vi "loadImageAndConvert.vi"(8 "error in (no error)":errorcluster, 10 "name or relative path":string) -> (0 "error out":errorcluster, 2 ".NET object":refnum<k24>)   [LabVIEW 2014, in "DataGrid.lvlib" / "DataTable.lvclass"]
uses:
  DataTable.lvclass
  System.Drawing
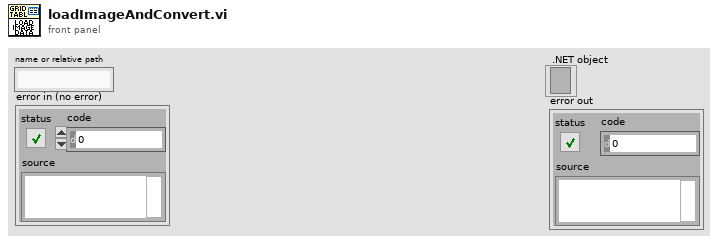
[diagram p1: front panel]
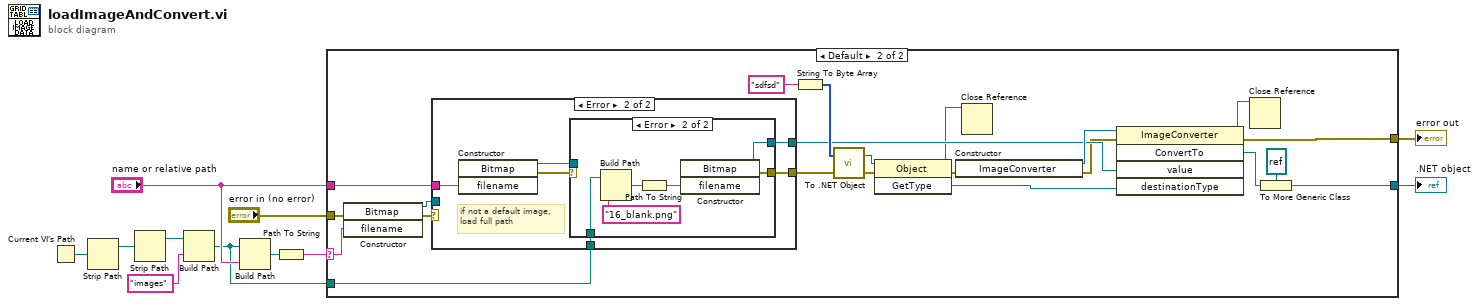
[diagram p0: block diagram]
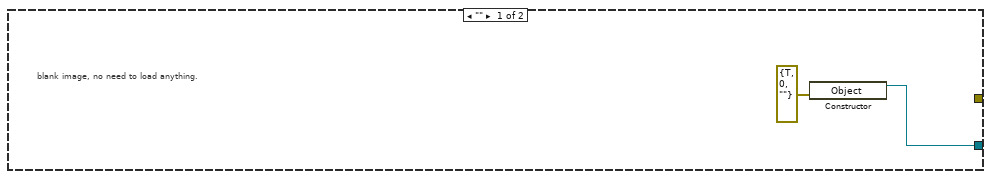
[diagram p2: hidden frame]
diagram:
  n1 = Current VI's Path() -> (path=w10:path)
  n2 = Strip Path(path=w10) -> (stripped path=w9:path)  [unwired: 1 out]
  n3 = Strip Path(path=w9) -> (stripped path=w7:path)  [unwired: 1 out]
  n4 = Build Path(base path=w7, name or relative path="images") -> (appended path=w1:path)
  n5 = Build Path(base path=w1, name or relative path="name or relative path") -> (appended path=w2:path)
  n6 = Path To String(path=w2) -> (string=w11:string)
  n7 = case shown="Default" w11 {
    selector: w11 -> [_ w35]
    tunnel: "name or relative path" -> [_ w33]
    tunnel: [w12 w16] -> w5
    tunnel: "error in (no error)" -> [_ w19]
    tunnel: [_ w15] -> w3
    tunnel: w1 -> [_ w14]
    frame "" {
      # "blank image, no need to load anything."
      n8 = constructor class="Object"(error in=errorcluster {"status"=TRUE, "code"=0, "source"=""} ("error in (no error)")) -> (reference out=w12:refnum<k24>)  [unwired: 2 in, 2 out]
    }
    frame Default {
      n9 = constructor class="Bitmap"(error in=w19, "filename"=w35) -> (reference out=w32:refnum<k24>, error out=w34:errorcluster)  [unwired: 2 in, 2 out]
      n10 = case shown="Error" w34 {
        tunnel: w33 -> [_ w42]
        tunnel: [w36 w40] -> w26
        tunnel: w32 -> [w36 _]
        tunnel: [_ w39] -> w23
        tunnel: w14 -> [_ w37]
        frame No Error {
          # "Used when a filename is given."
        }
        frame Error {
          # "if not a default image,\nload full path"
          n11 = constructor class="Bitmap"("filename"=w42) -> (reference out=w38:refnum<k24>, error out=w41:errorcluster)  [unwired: 3 in, 2 out]
          n12 = case shown="Error" w41 {
            selector: w41 -> [w43 _]
            tunnel: [w44 w50] -> w40
            tunnel: [w43 w49] -> w39
            tunnel: w38 -> [w44 _]
            tunnel: w37 -> [_ w45]
            frame No Error {
            }
            frame Error {
              n13 = Build Path(base path=w45, name or relative path="16_blank.png" ("filename")) -> (appended path=w48:path)
              n14 = Path To String(path=w48) -> (string=w47:string)
              n15 = constructor class="Bitmap"("filename"=w47) -> (reference out=w50:refnum<k24>, error out=w49:errorcluster)  [unwired: 3 in, 2 out]
            }
          }
        }
      }
      n16 = String To Byte Array(string="sdfsd") -> (unsigned byte array=w28:u8[])
      n17 = call <vilib>:"To .NET Object.vi"("error in (no error)"=w23, "anything"=w28) -> ("error out"=w22:errorcluster, ".NET object"=w29:refnum<k24>)
      n18 = invoke class="Object" method="GetType"(reference=w29, error in=w22) -> (reference out=w17:refnum<k24>, error out=w21:errorcluster, "GetType"=w30:refnum<k24>)  [unwired: 1 in]
      n19 = constructor class="ImageConverter"(error in=w21) -> (reference out=w27:refnum<k24>, error out=w20:errorcluster)  [unwired: 2 in, 1 out]
      n20 = Close Reference(reference=w17) -> ()  [unwired: 1 in, 1 out]
      n21 = invoke class="ImageConverter" method="ConvertTo"(reference=w27, error in=w20, "value"=w26, "destinationType"=w30) -> (reference out=w18:refnum<k24>, error out=w15:errorcluster, "ConvertTo"=w25:refnum<k24>)  [unwired: 1 in, 2 out]
      n22 = Close Reference(reference=w18) -> ()  [unwired: 1 in, 1 out]
      n23 = To More Generic Class(target class=refnum<k24> refnum (".NET object"), reference=w25) -> (generic class reference=w16:refnum<k24>)
    }
  }
  ".NET object" <- w5
  "error out" <- w3
